vi "Data Scaling Suite.vi"   [LabVIEW 2020, in "Unit Tests.lvlib"]
uses:
  Unit Tests.lvlib
  Tests/Data Scaling/Data Scaling.lvclass
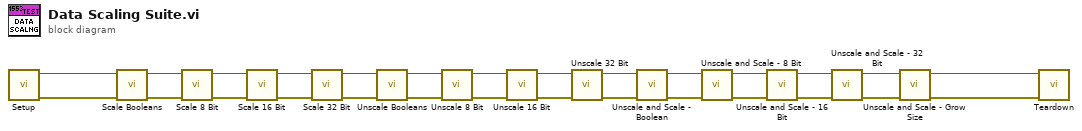
[diagram p0: block diagram]
diagram:
  n1 = call "Setup.vi"() -> ("error out"=w27:errorcluster, "Data Scaling out"=w28:refnum<class "Data Scaling.lvclass">)  [unwired: 10 in]
  n2 = call-dynamic "Scale Booleans.vi"("error in (no error)"=w27, "Data Scaling in"=w28) -> ("error out"=w17:errorcluster, "Data Scaling out"=w18:refnum<class "Data Scaling.lvclass">)  [unwired: 8 in]
  n3 = call-dynamic "Scale 8 Bit.vi"("error in (no error)"=w17, "Data Scaling in"=w18) -> ("error out"=w15:errorcluster, "Data Scaling out"=w16:refnum<class "Data Scaling.lvclass">)  [unwired: 8 in]
  n4 = call-dynamic "Scale 16 Bit.vi"("error in (no error)"=w15, "Data Scaling in"=w16) -> ("error out"=w13:errorcluster, "Data Scaling out"=w14:refnum<class "Data Scaling.lvclass">)  [unwired: 8 in]
  n5 = call-dynamic "Scale 32 Bit.vi"("error in (no error)"=w13, "Data Scaling in"=w14) -> ("error out"=w11:errorcluster, "Data Scaling out"=w12:refnum<class "Data Scaling.lvclass">)  [unwired: 8 in]
  n6 = call-dynamic "Unscale Booleans.vi"("error in (no error)"=w11, "Data Scaling in"=w12) -> ("error out"=w23:errorcluster, "Data Scaling out"=w24:refnum<class "Data Scaling.lvclass">)  [unwired: 8 in]
  n7 = call-dynamic "Unscale 8 Bit.vi"("error in (no error)"=w23, "Data Scaling in"=w24) -> ("error out"=w9:errorcluster, "Data Scaling out"=w10:refnum<class "Data Scaling.lvclass">)  [unwired: 8 in]
  n8 = call-dynamic "Unscale 16 Bit.vi"("error in (no error)"=w9, "Data Scaling in"=w10) -> ("error out"=w7:errorcluster, "Data Scaling out"=w8:refnum<class "Data Scaling.lvclass">)  [unwired: 8 in]
  n9 = call-dynamic "Unscale 32 Bit.vi"("error in (no error)"=w7, "Data Scaling in"=w8) -> ("error out"=w4:errorcluster, "Data Scaling out"=w6:refnum<class "Data Scaling.lvclass">)  [unwired: 8 in]
  n10 = call-dynamic "Unscale and Scale - Boolean.vi"("error in (no error)"=w4, "Data Scaling in"=w6) -> ("error out"=w3:errorcluster, "Data Scaling out"=w5:refnum<class "Data Scaling.lvclass">)  [unwired: 8 in]
  n11 = call-dynamic "Unscale and Scale - 8 Bit.vi"("error in (no error)"=w3, "Data Scaling in"=w5) -> ("error out"=w19:errorcluster, "Data Scaling out"=w21:refnum<class "Data Scaling.lvclass">)  [unwired: 8 in]
  n12 = call-dynamic "Unscale and Scale - 16 Bit.vi"("error in (no error)"=w19, "Data Scaling in"=w21) -> ("error out"=w20:errorcluster, "Data Scaling out"=w22:refnum<class "Data Scaling.lvclass">)  [unwired: 8 in]
  n13 = call-dynamic "Unscale and Scale - 32 Bit.vi"("error in (no error)"=w20, "Data Scaling in"=w22) -> ("error out"=w1:errorcluster, "Data Scaling out"=w2:refnum<class "Data Scaling.lvclass">)  [unwired: 8 in]
  n14 = call-dynamic "Unscale and Scale - Grow Size.vi"("error in (no error)"=w1, "Data Scaling in"=w2) -> ("error out"=w25:errorcluster, "Data Scaling out"=w26:refnum<class "Data Scaling.lvclass">)  [unwired: 8 in]
  n15 = call-dynamic "Teardown.vi"("error in (no error)"=w25, "Data Scaling in"=w26) -> ()  [unwired: 9 in, 1 out]
